vi "destroyEvent.vi"(8 "error in (no error)":errorcluster, 11 "Handler.UserEvent.Console in":refnum<class "Handler.UserEvent.Console.lvclass">) -> (0 "error out":errorcluster, 3 "Handler.UserEvent.Console out":refnum<class "Handler.UserEvent.Console.lvclass">)   [LabVIEW 2017, in "Error Log.lvlib" / "Handler.UserEvent.Console.lvclass"]
uses:
  Handler.UserEvent.Console.lvclass
  Handler.UserEvent.Console.lvclass/Handler.UserEvent.Console.ctl
  Handler.UserEvent/Handler.UserEvent.lvclass
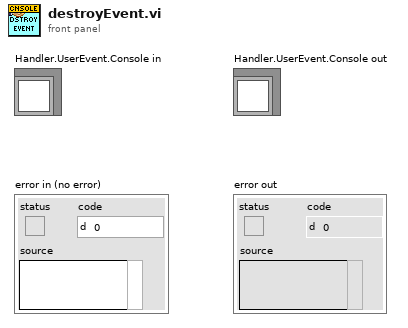
[diagram p1: front panel]
types:
  T1 = typedef "Error Log.lvlib/Handler.UserEvent.Console.lvclass/privateEvents.ctl" = cluster{"Stop":refnum<user-event>, "Show Hide UI":refnum<user-event>, "Clear":refnum<user-event>}
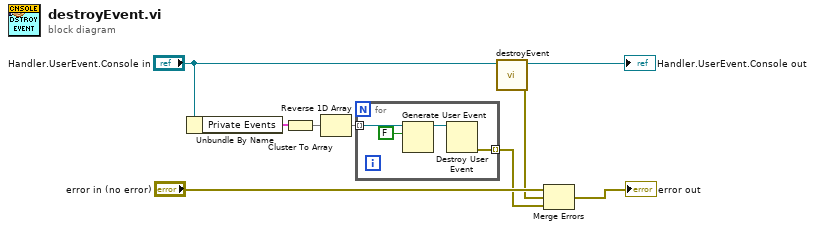
[diagram p0: block diagram]
diagram:
  n1 = Unbundle By Name("Handler.UserEvent.Console in") -> ("Private Events"=w9:T1)
  n2 = Cluster To Array(cluster=w9) -> (array=w8:refnum<user-event>[])
  n3 = Reverse 1D Array(array=w8) -> (reversed array=w1:refnum<user-event>[])
  n4 = for {
    tunnel: w1 -> [w13] mode=indexing
    tunnel: [w12] -> w4 mode=indexing
    n5 = Generate User Event(user event=w13, event data cluster=FALSE ("event data")) -> (user event out=w11:refnum<user-event>)  [unwired: 2 in, 1 out]
    n6 = Destroy User Event(user event=w11) -> (error out=w12:errorcluster)  [unwired: 1 in]
  }
  n7 = call-parent "destroyEvent.vi"("Handler.UserEvent in"="Handler.UserEvent.Console in") -> ("error out"=w5:errorcluster, "Handler.UserEvent out"=→"Handler.UserEvent.Console out":refnum<class "Handler.UserEvent.Console.lvclass">)  [unwired: 9 in]
  n8 = Merge Errors("error in (no error)", w5, w4) -> (→"error out":errorcluster)
